vi "inputGetParameter.vi"() -> (1 "Device Parameter":u8[](array[numeric]), 2 "a_pNumPixelsInput":u16)   [LabVIEW 2016]
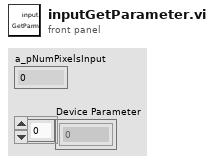
[diagram p1: front panel]
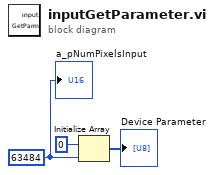
[diagram p0: block diagram]
diagram:
  w2 = u16 63484 ("a_pNumPixelsInput")
  n1 = Initialize Array(u8 0, w2) -> (→"Device Parameter":u8[])
  "a_pNumPixelsInput" <- w2
